vi "TSM Sync Initialize Sessions.vi"(0 "TSM context":T1) -> (15 "error out":errorcluster)   [LabVIEW 2019]
doc: "Use this VI to initialize sessions for all NI-SYNC instruments in the pin map associated with the test program."
uses:
  <vilib>/NI_TestStand_SemiconductorModule/NI_TestStand_Semiconductor_Module.lvlibp/PinMap/General/SemiconductorModuleContext.ctl
  <instrlib>/niSync/niSync.llb/niSync Initialize (Default).vi
  <vilib>/NI_TestStand_SemiconductorModule/NI_TestStand_Semiconductor_Module.lvlibp
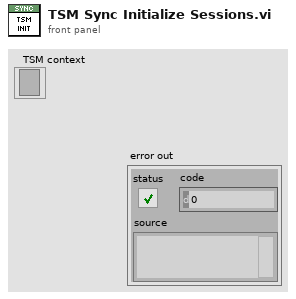
[diagram p1: front panel]
types:
  T1 = typedef "NI_TestStand_Semiconductor_Module.lvlibp/SemiconductorModuleContext.ctl" = refnum<k7>
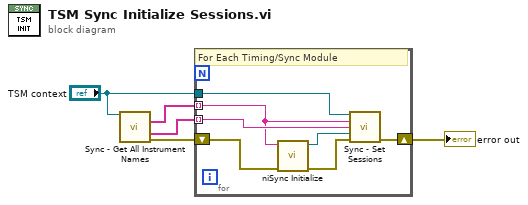
[diagram p0: block diagram]
diagram:
  n1 = call "Sync - Get All Instrument Names.vi"("TSM context"="TSM context") -> ("Instrument Names"=w5:string[], "Channel Group Ids"=w4:string[], "error out"=w3:errorcluster)  [unwired: 10 in, 2 out]
  n2 = for {
    tunnel: w5 -> [w6] mode=indexing
    tunnel: "TSM context" -> [w11]
    tunnel: w4 -> [w10] mode=indexing
    shift-right: [w12] -> w2
    shift-left: w3 -> [w8]
    # "For Each Timing/Sync Module"
    n3 = call-poly <instrlib>:"niSync Initialize.vi"("error in (no error)"=w8, "resource name"=w6) -> ("error out"=w9:errorcluster, "instrument handle out"=w7:refnum<k15>)  [unwired: 8 in]
    n4 = call "Sync - Set Sessions.vi"("TSM context"=w11, "Instrument Name"=w6, "Channel Group  Id"=w10, "Sync Session"=w7, "error in"=w9) -> ("error out"=w12:errorcluster)  [unwired: 9 in, 1 out]
  }
  "error out" <- w2
